vi "BaseClassDependencyGetter.vi"(8 "error in (no error)":errorcluster, 11 "Level2Class in":refnum<class "Level2Class.lvclass">) -> (0 "error out":errorcluster, 1 "BaseClassDependency out":refnum<class "BaseClassDependency.lvclass">, 3 "Level2Class out":refnum<class "Level2Class.lvclass">)   [LabVIEW 2019, in "Level2Class.lvlib" / "Level2Class.lvclass"]
uses:
  Level2Class.lvclass
  BaseClassDependency/BaseClassDependency.lvclass
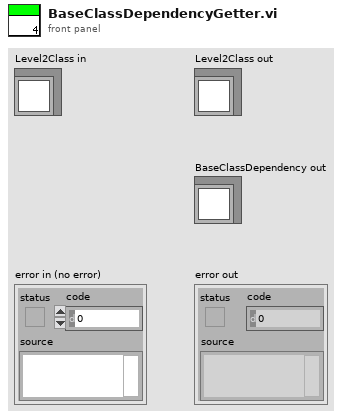
[diagram p1: front panel]
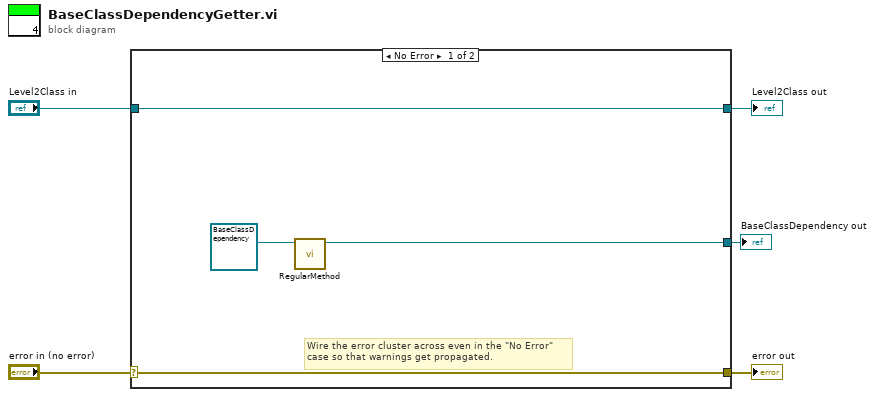
[diagram p0: block diagram]
diagram:
  n1 = case shown="No Error" "error in (no error)" {
    selector: "error in (no error)" -> [w8 w11]
    tunnel: [w8 w11] -> w4
    tunnel: [w9 w10] -> w2
    tunnel: "Level2Class in" -> [w9 w10]
    tunnel: [w6 _] -> w1
    frame No Error {
      # "Wire the error cluster across even in the \"No Error\"\ncase so that warnings get propagated."
      n2 = call-dynamic "RegularMethod.vi"("BaseClassDependency in"=refnum<class "BaseClassDependency.lvclass"> refnum ("BaseClassDependency.lvlib:BaseClassDependency.lvclass")) -> ("BaseClassDependency out"=w6:refnum<class "BaseClassDependency.lvclass">)  [unwired: 9 in, 1 out]
    }
    frame Error {
    }
  }
  "error out" <- w4
  "Level2Class out" <- w2
  "BaseClassDependency out" <- w1
